vi "WGS_Query.vi"(0 "System no.":i32=1 min=1 max=4 step=1, 2 "WaveGeneratorID":i32=-1, 3 "Item":string, 4 "Query all?":bool=TRUE, 5 "error in":errorcluster) -> (14 "Value (num.)":dbl[](array[numeric]) format="%.6f", 15 "Value (string)":string[](array[string]), 16 "WaveGeneratorID out":i32[](array[numeric]), 17 "Item out":string[](array[string]), 19 "error out":errorcluster)   [LabVIEW 2020]
doc: "Get status information of wave generator.\n\nIf Query all? = FALSE, a valid wave generator ID has to be specified.\n\nItem is only taken into account if Query all? = FALSE and a valid wave generator ID has been specified. If Item is an empty string, all items of the given wave generator ID are queried."
panel:
  # "Get status information of wave generator."
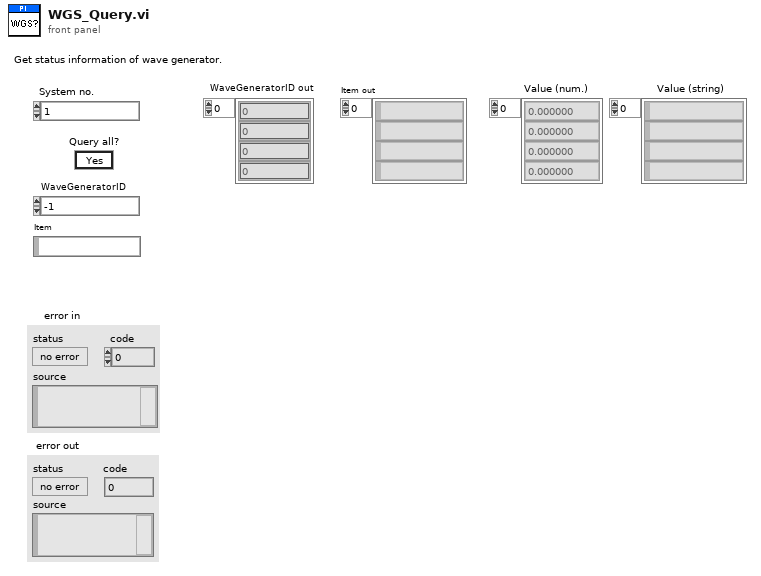
[diagram p1: front panel]
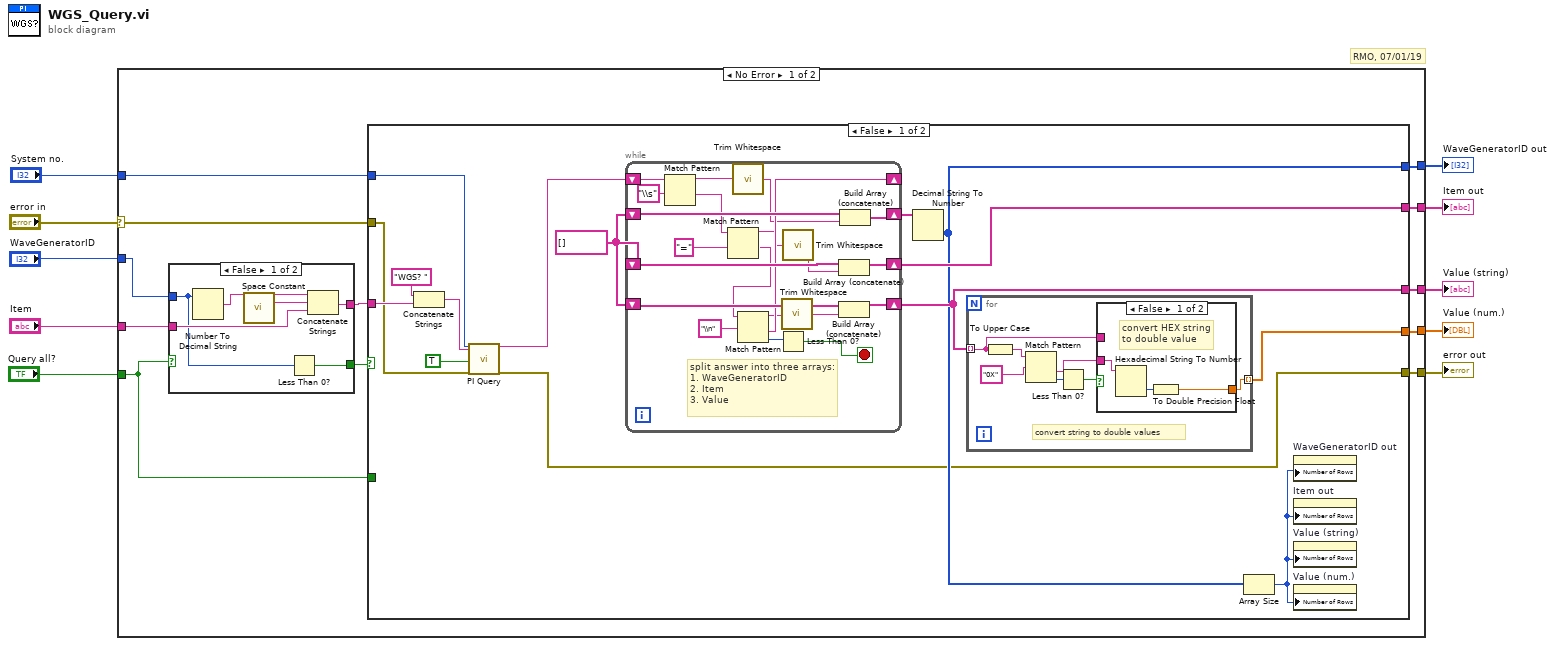
[diagram p0: block diagram]
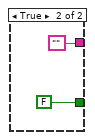
[diagram p2: hidden frame]
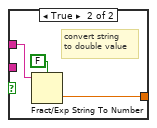
[diagram p3: hidden frame]
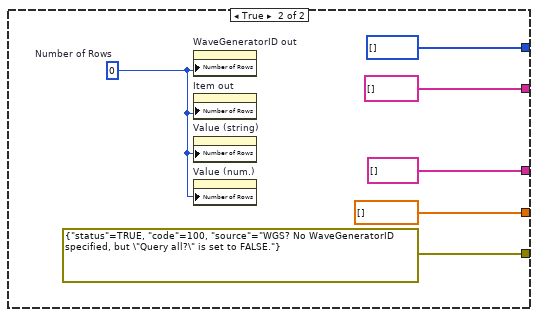
[diagram p4: hidden frame]
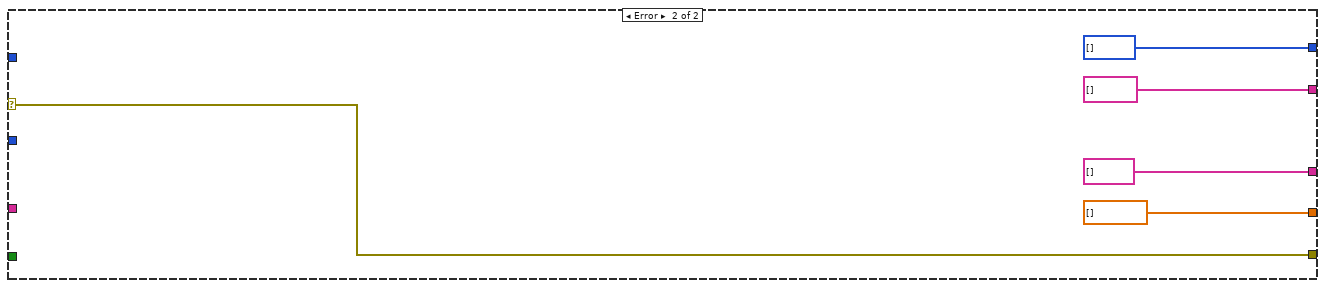
[diagram p5: hidden frame]
diagram:
  # "RMO, 07/01/19"
  n1 = case shown="No Error" "error in" {
    selector: "error in" -> [w11 w86]
    tunnel: "Item" -> [w12 _]
    tunnel: "System no." -> [w16 _]
    tunnel: "WaveGeneratorID" -> [w21 _]
    tunnel: [w20 w86] -> w7
    tunnel: [w18 dbl[] [] ("Parameter values")] -> w6
    tunnel: "Query all?" -> [w13 _]
    tunnel: [w17 string[] [] ("Parameter strings")] -> w5
    tunnel: [w15 string[] [] ("Queried axes out")] -> w4
    tunnel: [w14 i32[] [] ("Parameter no. out")] -> w3
    frame No Error {
      n2 = case shown="False" w13 {
        tunnel: w12 -> [w26 _]
        tunnel: [w27 "" ("Command substring")] -> w22
        tunnel: w21 -> [w23 _]
        tunnel: [w24 FALSE] -> w19
        frame False {
          n3 = Number To Decimal String(number=w23) -> (decimal integer string=w25:string)  [unwired: 1 out]
          n4 = call "Space Constant.vi"() -> ("String"=w28:string)
          n5 = Less Than 0?(x=w23) -> (x < 0?=w24:bool)
          n6 = Concatenate Strings(w25, w28, w26) -> (w27:string)
        }
        frame True {
        }
      }
      n7 = case shown="False" w19 {
        tunnel: w11 -> [w42 _]
        tunnel: w22 -> [w43 _]
        tunnel: w16 -> [w41 _]
        tunnel: [w32 errorcluster {"status"=TRUE, "code"=100, "source"="WGS? No WaveGeneratorID specified, but \"Query all?\" is set to FALSE."} ("error out")] -> w20
        tunnel: [w35 dbl[] [] ("Parameter values")] -> w18
        tunnel: [w36 string[] [] ("Parameter strings")] -> w17
        tunnel: [w38 string[] [] ("Queried axes out")] -> w15
        tunnel: [w34 i32[] [] ("Parameter no. out")] -> w14
        tunnel: w13 -> [_ _]
        frame False {
          w40 = string[] []
          n8 = Concatenate Strings("WGS? ", w43) -> (w44:string)
          n9 = call "PI Query.vi"("System no."=w41, "String to send"=w44, "Attach termination char.?"=TRUE ("Attach Linefeed?"), "error in"=w42) -> ("String read"=w31:string, "error out"=w32:errorcluster)  [unwired: 3 in, 11 out]
          n10 = while {
            shift-right: [w66] -> _
            shift-left: w31 -> [w79]
            shift-right: [w76] -> w39
            shift-left: w40 -> [w77]
            shift-right: [w74] -> w38
            shift-left: w40 -> [w75]
            shift-right: [w72] -> w36
            shift-left: w40 -> [w73]
            stop <- w59 stop-if-true
            # "split answer into three arrays:\n1. WaveGeneratorID\n2. Item\n3. Value"
            n11 = Match Pattern(string=w79, regular expression="\\s") -> (before substring=w65:string, after substring=w68:string)  [unwired: 3 out]
            n12 = Match Pattern(string=w68, regular expression="=") -> (before substring=w63:string, after substring=w67:string)  [unwired: 3 out]
            n13 = call "Trim Whitespace.vi"("string"=w65) -> ("trimmed string"=w64:string)  [unwired: 1 in]
            n14 = Match Pattern(string=w67, regular expression="\\n") -> (before substring=w60:string, after substring=w66:string, offset past match=w69:i32)  [unwired: 2 out]
            n15 = Less Than 0?(x=w69) -> (x < 0?=w59:bool)
            n16 = call "Trim Whitespace.vi"("string"=w60) -> ("trimmed string"=w61:string)  [unwired: 1 in]
            n17 = call "Trim Whitespace.vi"("string"=w63) -> ("trimmed string"=w62:string)  [unwired: 1 in]
            n18 = Build Array (concatenate)(w75, w62) -> (w74:string[])
            n19 = Build Array (concatenate)(w73, w61) -> (w72:string[])
            n20 = Build Array (concatenate)(w77, w64) -> (w76:string[])
          }
          n21 = Decimal String To Number(string=w39) -> (number=w34:i32[])  [unwired: 3 out]
          n22 = for {
            tunnel: w36 -> [w46] mode=indexing
            tunnel: [w47] -> w35 mode=indexing
            # "convert string to double values"
            n23 = To Upper Case(1:w46) -> (0:w52:string)
            n24 = Match Pattern(string=w52, regular expression="0X") -> (after substring=w48:string, offset past match=w50:i32)  [unwired: 3 out]
            n25 = Less Than 0?(x=w50) -> (x < 0?=w49:bool)
            n26 = case shown="False" w49 {
              tunnel: w48 -> [w55 _]
              tunnel: [w53 w57] -> w47
              tunnel: w46 -> [_ w56]
              frame False {
                # "convert HEX string\nto double value"
                n27 = Hexadecimal String To Number(string=w55) -> (number=w54:u32)  [unwired: 3 out]
                n28 = To Double Precision Float(number=w54) -> (double precision float=w53:dbl)
              }
              frame True {
                # "convert string\nto double value"
                n29 = Fract/Exp String To Number(use system decimal point (T)=FALSE, string=w56) -> (number=w57:dbl)  [unwired: 3 out]
              }
            }
          }
          n30 = Array Size(array=w34) -> (size(s)=w37:i32)
          n31 = property on="WaveGeneratorID out" class="Arr (strict)"("Number of Rows"=w37) -> ()  [unwired: 2 in, 2 out]
          n32 = property on="Item out" class="Arr (strict)"("Number of Rows"=w37) -> ()  [unwired: 2 in, 2 out]
          n33 = property on="Value (string)" class="Arr (strict)"("Number of Rows"=w37) -> ()  [unwired: 2 in, 2 out]
          n34 = property on="Value (num.)" class="Arr (strict)"("Number of Rows"=w37) -> ()  [unwired: 2 in, 2 out]
        }
        frame True {
          w80 = u32 0  # Number of Rows
          n35 = property on="WaveGeneratorID out" class="Arr (strict)"("Number of Rows"=w80) -> ()  [unwired: 2 in, 2 out]
          n36 = property on="Item out" class="Arr (strict)"("Number of Rows"=w80) -> ()  [unwired: 2 in, 2 out]
          n37 = property on="Value (string)" class="Arr (strict)"("Number of Rows"=w80) -> ()  [unwired: 2 in, 2 out]
          n38 = property on="Value (num.)" class="Arr (strict)"("Number of Rows"=w80) -> ()  [unwired: 2 in, 2 out]
        }
      }
    }
    frame Error {
    }
  }
  "error out" <- w7
  "Value (num.)" <- w6
  "Value (string)" <- w5
  "Item out" <- w4
  "WaveGeneratorID out" <- w3
